vi "ConfigureRF.vi"(8 "error in (no error)":errorcluster, 11 "reference in":refnum<class "niMmWave_Reciever.lvclass">) -> (0 "error out":errorcluster, 3 "reference out":refnum<class "niMmWave_Reciever.lvclass">)   [LabVIEW 2019, in "niMmWave_Reciever.lvclass"]
doc: "Configures RF setting at specified port:\n<b>Frequency</b> - operating frequency (RF/IF)\n<b>Gain</b> - Signal gain"
uses:
  niMmWave_Reciever.lvclass
  C:/Barkhausen mmWave radar/Development/modules/mmw_instrument/src_LabVIEW/Host/SubVIs/mmWave instrument_class/mmWave instrument.lvclass
  Low-level/TypeDefs/Front End Configuration.ctl
  Low-level/TypeDefs/Channel Configuration.ctl
  <instrlib>/niMmWave/ni3620/Config/v1/Host/Public/Typedefs/mmWave Port.ctl
  mmWave instrument_class/mmWave instrument.lvclass
  mmWave HW Control/mmWave HW Control.lvlib
  <instrlib>/niMmWave/ni3620/Config/v1/Host/niMmWave Config v1 Host.lvlib
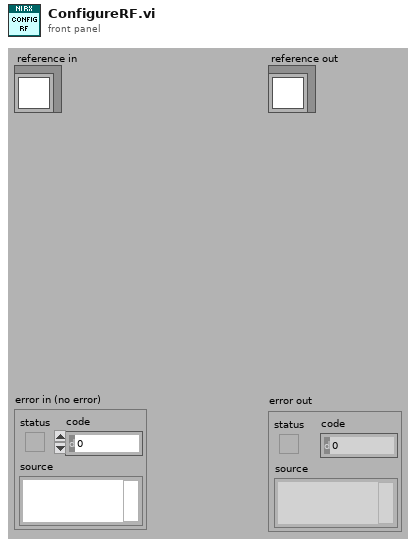
[diagram p1: front panel]
types:
  T1 = typedef "niMmWave Config v1 Host.lvlib/mmWave Port.ctl" = string
  T2 = typedef "Front End Configuration.ctl" = cluster{"port select":enum16{"IF Port", "Loopback", "Sync Port"}, "Rx hardware configuration":T3, "Tx hardware configuration":T3}
  T3 = typedef "Channel Configuration.ctl" = cluster{"gain (dB)":dbl, "frequency (Hz)":dbl, "mmWave adapter":string, "adapter active port":T1}
  T4 = typedef "niMmWave_Reciever.lvclass/ObjectAttributesRef.ctl" = refnum<data-value>
  T5 = typedef "mmWave instrument.lvclass/ObjectAttributes.ctl" = cluster{"mode":T6, "instr state":T7, "Max Fs":dbl, "Equalization coeff":cdb[], "LO sync en":bool, "Trig sync en":bool, "LO sources":T8, "LO Export":T9, "Fc.range":cluster{"min":dbl, "max":dbl}, "Sync mode":T10, "equalization en":bool, "sequence":string[]}
  T6 = typedef "mmWave instrument.lvclass/Instrument mode.ctl" = enum16{"RF", "IF", "BB"}
  T7 = typedef "mmWave instrument.lvclass/Instrument state.ctl" = enum16{"Off", "Initialization", "Configuration", "Running", "Calibration"}
  T8 = typedef "mmWave HW Control.lvlib/LO sources.ctl" = cluster{"RX/LO1 src":string, "TX/LO1 src":string, "LO2 src":string}
  T9 = typedef "mmWave HW Control.lvlib/LO export.ctl" = cluster{"TX LO1 export":bool, "TX LO1 export level":dbl, "RX LO1 export":bool, "RX LO1 export level":dbl, "LO2 export":bool, "LO2 export level":dbl}
  T10 = typedef "mmWave instrument.lvclass/Sync mode.ctl" = enum16{"Slave", "Master"}
  T11 = typedef "niMmWave_Reciever.lvclass/ObjectAttributes.ctl" = cluster{"session":T12[], "HW.RX devices":T26, "RF config":T27, "RX trigger options":T28, "RX samples":i32, "RX Fs":dbl}
  T12 = typedef "Session.ctl" = cluster{"3620 session":refnum<queue>, "tx baseband session":T13, "rx baseband session":T21, "tx gain (dB)":dbl, "rx gain (dB)":dbl, "hardware configuration":T22, "gain ranging":T24[], "pxi trigger bus information":T25}
  T13 = typedef "Tx Baseband Session.ctl" = cluster{"3610 session":T14, "7902 reference":T20}
  T14 = typedef "ni3610_and_ni3630_Driver_Lib.lvlib/Main Settings.ctl" = cluster{"VISA resource name":refnum<visa-resource-name>, "Address Space":T15, "window_offset":u32, "register_addresses":T16, "required_MM_fpga_version":cluster{"signature":u32, "hardware":u32, "current revision":u32, "oldest revision":u32}, "CPLD Oldest Compat Version ":cluster{"hardware":u32, "CPLD firmware":u32}, "MM_FPGA_image_location":string, "is_init":bool, "card_type":T17, "DacLmkConfigFileName":string, "AdcLmkConfigFileName":string, "AdcConfigFileName":string, "DacConfigFileName_RevA":string, "DacConfigFileName_RevB":string, "Mulde hardware revision":u8, "bypass DAC PLL\n":bool, "IQ Card Revision":T18, "board capability":T19}
  T15 = typedef "VISA Register Access Address Space.ctl" = u16
  T16 = typedef "ni3610_and_ni3630_Driver_Lib.lvlib/Register Adresses.ctl" = cluster{"MM based Registers":cluster{"Revision":u32, "OldestCompatRev":u32, "signature":u32, "scratch":u32, "LedControl":u32, "BoardHwRev":u32, "BoardControl":u32, "ThermalStatus":u32, "BasebandStatus":u32, "BasebandControl":u32, "BasebandAuxSetup":u32, "BasebandAuxStatus":u32, "LmkSyncOutSetup":u32, " AdcSyncOutSetup":u32, " InjSyncOutSetup":u32, " PxiTrig0OutSetup":u32, " PxiTrig1OutSetup":u32, " PxiTrig2OutSetup":u32, " PxiTrig3OutSetup":u32, " PxiTrig4OutSetup":u32, " PxiTrig5OutSetup":u32, " PxiTrig6OutSetup":u32, " PxiTrig7OutSetup":u32}, "CPLD based Registers":cluster{"SlaveSignature":u32, "SlaveRevision":u32, "SlaveOldestCompatRev":u32, "SlaveScratch":u32, "SlaveSetup":u32, "SlaveStatus":u32, "IDacReg_offset":u32, "LMKRegGrp0_offset":u32, "QDacReg_offset":u32, "BrdTempSensorVal":u32, "TempSensorPowerDown":u32, "GPIOReg_offset":u32, "IAdcReg_offset":u32, "QAdcReg_offset":u32, "LMKRegGrp1_offset":u32, "QadcTempSensorVal":u32, "IadcTempSensorVal":u32, "RevisionReg":u32, "VcxoReg":u32, "CpldStatusReg":u32, "PowerReg":u32, "VBiasEnReg":u32, "ExtRefOeReg":u32, "QdacCtrlReg":u32, "QdacStatusReg":u32, "IdacCtrlReg":u32, "IdacStatusReg":u32, "QdacJtagIn":u32, "QdacJtagOut":u32, "IdacJtagIn":u32, "IdacJtagOut":u32, "IqDcSetupReg":u32, "QadcStatusReg":u32, "IadcStatusReg":u32, "BrdSetupReg":u32, "IqDcRevisionReg":u32, "PllStatusReg":u32, "EndpointScratchReg":u32, "AdcSyncCfgReg":u32, "IqCardOpampReg":u32}, "CPLD Register Offset":u32, "MM  Register Offset":u32, " PxiTrig0OutSetup":u32}
  T17 = typedef "ni3610_and_ni3630_Driver_Lib.lvlib/Base Card Type.ctl" = enum16{"unspecified", "ADC", "DAC"}
  T18 = typedef "ni3610_and_ni3630_Driver_Lib.lvlib/IQ Card Revision.ctl" = enum16{"RevA", "RevB", "RevC", "RevD"}
  T19 = typedef "ni3610_and_ni3630_Driver_Lib.lvlib/Board Capability.ctl" = cluster{"baseband sync":enum16{"no baseband sync", "baseband sync"}}
  T20 = typedef "Blank FPGA Reference.ctl" = refnum<k20>
  T21 = typedef "Rx Baseband Session.ctl" = cluster{"3630 session":T14, "7902 reference":T20}
  T22 = typedef "Hardware Configuration.ctl" = cluster{"direction":T23, "baseband only":bool}
  T23 = typedef "Direction.ctl" = enum16{"Transceiver", "Receiver", "Transmitter"}
  T24 = typedef "Gain Ranging.ctl" = cluster{"gain ranging active scope":string, "gain ranging stream session":refnum<k20>}
  T25 = typedef "PXI Trigger Bus Info.ctl" = cluster{"chassis resource name":refnum<visa-resource-name>, "7902R (TX)":i16, "3610 (TX)":i16, "3620 (IF)":i16, "3630 (RX)":i16, "7902R (RX)":i16}
  T26 = typedef "mmWave HW Control.lvlib/HW RX resources cluster.ctl" = cluster{"HW.IF":tag, "HW.ADC":refnum<visa-resource-name>, "HW.RX FPGA":tag}
  T27 = typedef "mmWave HW Control.lvlib/HW RX RF config cluster.ctl" = cluster{"Gain":dbl, "Frequency":dbl, "mmWave adapter":string}
  T28 = typedef "TX trigger config.ctl" = cluster{"delay":dbl, "trig source":T29, "PXI src":i32, "export":T30, "PXI dest":i32}
  T29 = typedef "FPGA Utility.lvlib/FPGA driver trigger source.ctl" = enum16{"Use Tclk", "PXI_Trig", "Aurora RX trig"}
  T30 = typedef "FPGA Utility.lvlib/FPGA driver trigger destination.ctl" = enum16{"None", "Source trig", "Synced trig", "Delayed sync"}
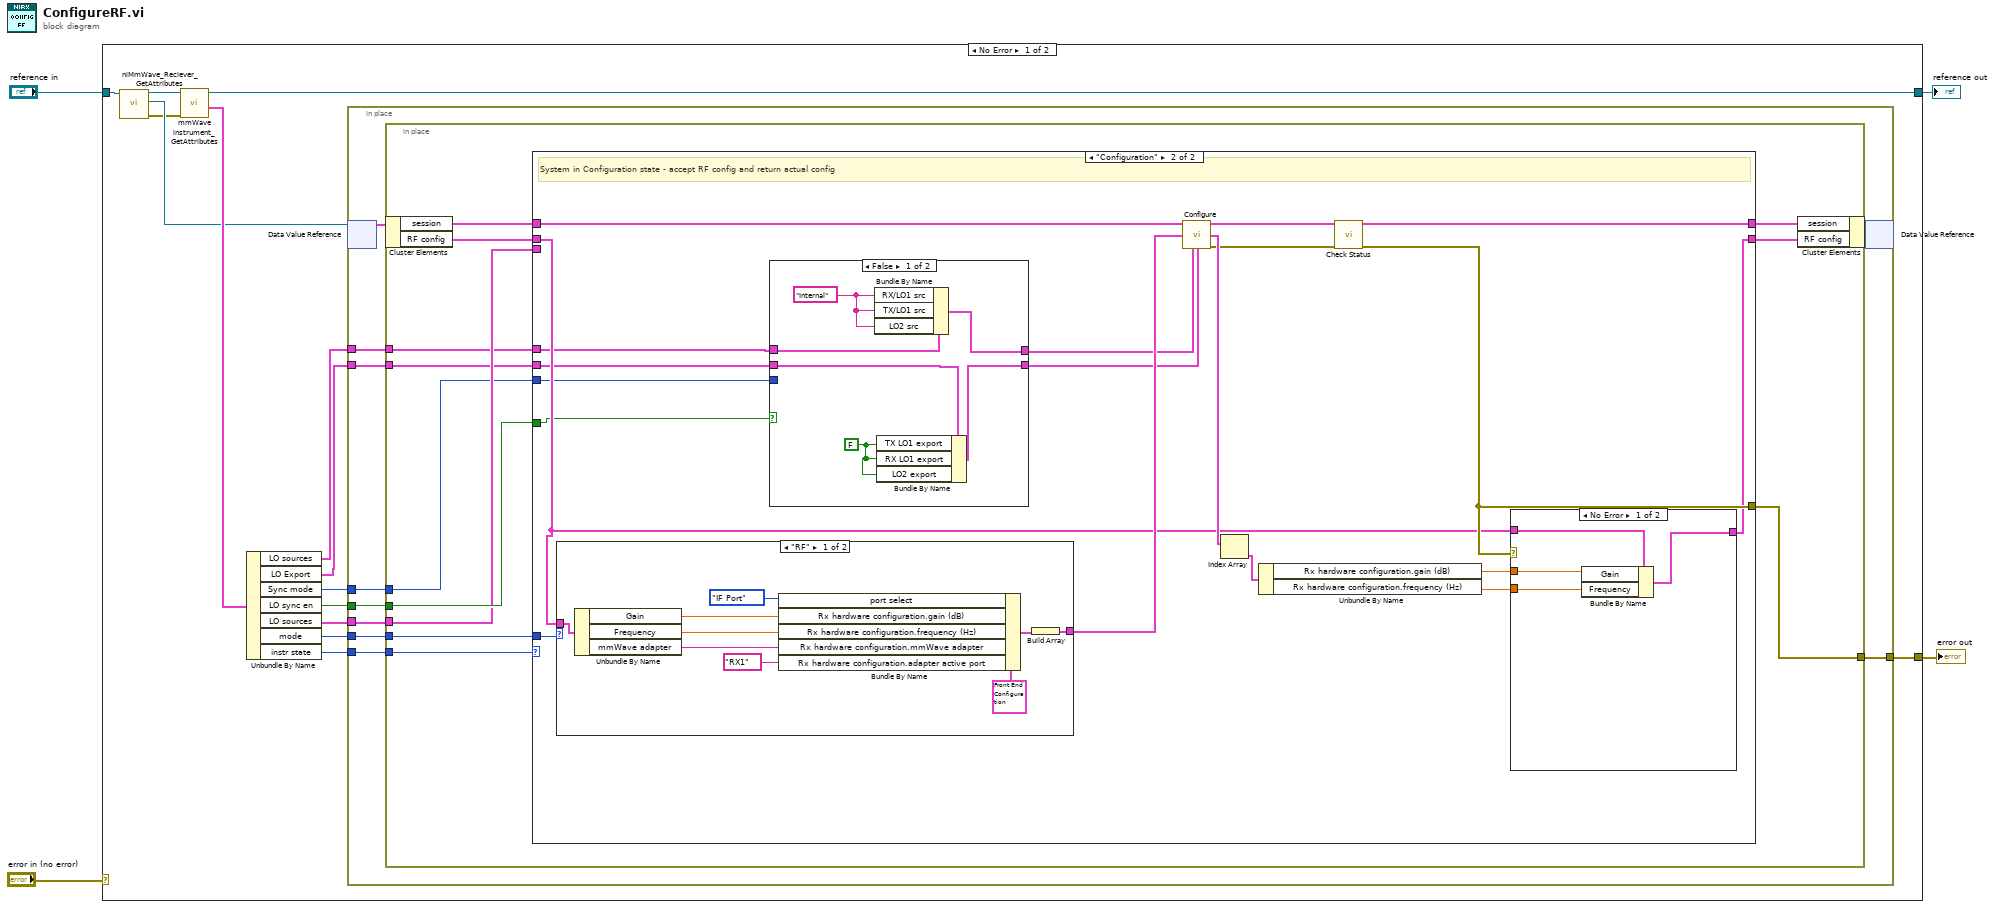
[diagram p0: block diagram]
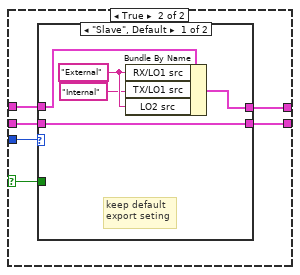
[diagram p3: hidden frame]
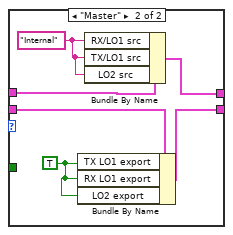
[diagram p4: hidden frame]
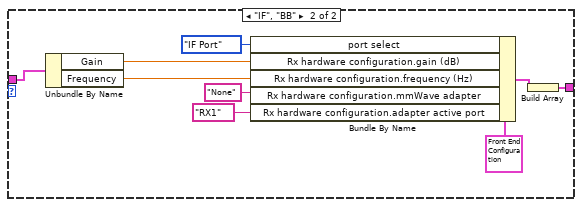
[diagram p6: hidden frame]
diagram:
  n1 = case shown="No Error" "error in (no error)" {
    selector: "error in (no error)" -> [_ w109]
    tunnel: [w12 w109] -> w3
    tunnel: [w16 w108] -> w1
    tunnel: "reference in" -> [w17 w108]
    frame No Error {
      n2 = call "niMmWave_Reciever_GetAttributes.vi"("reference in"=w17) -> ("error out"=w13:errorcluster, "attributes ref"=w14:T4, "reference out"=w18:refnum<class "niMmWave_Reciever.lvclass">)  [unwired: 7 in, 1 out]
      n3 = call "mmWave instrument_GetAttributes.vi"("error in (no error)"=w13, "reference in"=w18) -> ("attributes"=w15:T5, "reference out"=w16:refnum<class "niMmWave_Reciever.lvclass">)  [unwired: 6 in, 2 out]
      n4 = Unbundle By Name(w15) -> ("LO sources"=w7:T8, "LO Export"=w6:T9, "Sync mode"=w5:T10, "LO sync en"=w9:bool, "LO sources"=w8:T8, "mode"=w11:T6, "instr state"=w10:T7)
      n5 = in-place {
        in-place-border: [w27] -> w12
        in-place-border: w11 -> [w26]
        in-place-border: w10 -> [w25]
        in-place-border: w9 -> [w23]
        in-place-border: w8 -> [w22]
        in-place-border: w7 -> [w21]
        in-place-border: w6 -> [w20]
        in-place-border: w5 -> [w19]
        n6 = in-place-dvr #1(w14) -> (w24:T11)  [unwired: 1 out]
        n7 = in-place {
          in-place-border: [w37] -> w27
          in-place-border: w26 -> [w38]
          in-place-border: w25 -> [w35]
          in-place-border: w23 -> [w33]
          in-place-border: w22 -> [w32]
          in-place-border: w21 -> [w31]
          in-place-border: w20 -> [w30]
          in-place-border: w19 -> [w29]
          n8 = in-place-cluster #2(w24) -> ("session"=w40:T12[], "RF config"=w34:T27)
          n9 = case shown="\"Configuration\"" w35 {
            tunnel: w40 -> [w42 w60]
            tunnel: [w42 w59] -> w39
            tunnel: w38 -> [_ w58]
            tunnel: [_ w55] -> w37
            tunnel: [w41 w52] -> w36
            tunnel: w34 -> [w41 w51]
            tunnel: w33 -> [_ w46]
            tunnel: w32 -> [_ _]
            tunnel: w31 -> [_ w47]
            tunnel: w30 -> [_ w45]
            tunnel: w29 -> [_ w43]
            frame "Off", Default {
            }
            frame "Configuration" {
              # "System in Configuration state - accept RF config and return actual config"
              n10 = case shown="\"RF\"" w58 {
                tunnel: [w98 w107] -> w61
                tunnel: w51 -> [w93 w102]
                frame "RF" {
                  n11 = Unbundle By Name(w93) -> ("Gain"=w92:dbl, "Frequency"=w91:dbl, "mmWave adapter"=w90:string)
                  n12 = Bundle By Name(cluster=T2 {"port select"=enum."Loopback", "Rx hardware configuration"={"gain (dB)"=15.0, "frequency (Hz)"=12000000000.0, "mmWave adapter"="None", "adapter active port"=""}, "Tx hardware configuration"={"gain (dB)"=-15.0, "frequency (Hz)"=12000000000.0, "mmWave adapter"="None", "adapter active port"=""}} ("device configuration [channel]"), "port select"=enum16{"IF Port", "Loopback", "Sync Port"}."IF Port", "Rx hardware configuration.gain (dB)"=w92, "Rx hardware configuration.frequency (Hz)"=w91, "Rx hardware configuration.mmWave adapter"=w90, "Rx hardware configuration.adapter active port"=T1 "RX1") -> (w97:T2)
                  n13 = Build Array(w97) -> (w98:T2[])
                }
                frame "IF", "BB" {
                  n14 = Unbundle By Name(w102) -> ("Gain"=w101:dbl, "Frequency"=w100:dbl)
                  n15 = Bundle By Name(cluster=T2 {"port select"=enum."Loopback", "Rx hardware configuration"={"gain (dB)"=15.0, "frequency (Hz)"=12000000000.0, "mmWave adapter"="None", "adapter active port"=""}, "Tx hardware configuration"={"gain (dB)"=-15.0, "frequency (Hz)"=12000000000.0, "mmWave adapter"="None", "adapter active port"=""}} ("device configuration [channel]"), "port select"=enum16{"IF Port", "Loopback", "Sync Port"}."IF Port", "Rx hardware configuration.gain (dB)"=w101, "Rx hardware configuration.frequency (Hz)"=w100, "Rx hardware configuration.mmWave adapter"="None", "Rx hardware configuration.adapter active port"=T1 "RX1") -> (w106:T2)
                  n16 = Build Array(w106) -> (w107:T2[])
                }
              }
              n17 = case shown="False" w46 {
                selector: w46 -> [_ w68]
                tunnel: w47 -> [w67 w69]
                tunnel: w45 -> [w63 w73]
                tunnel: [w66 w70] -> w48
                tunnel: [w62 w72] -> w44
                tunnel: w43 -> [_ w71]
                frame False {
                  w64 = FALSE
                  w65 = "Internal" ("RX/LO1 src")
                  n18 = Bundle By Name(cluster=w67, "RX/LO1 src"=w65, "TX/LO1 src"=w65, "LO2 src"=w65) -> (w66:T8)
                  n19 = Bundle By Name(cluster=w63, "TX LO1 export"=w64, "RX LO1 export"=w64, "LO2 export"=w64) -> (w62:T9)
                }
                frame True {
                  n20 = case shown="\"Slave\", Default" w71 {
                    tunnel: w73 -> [w75 w84]
                    tunnel: [w75 w83] -> w72
                    tunnel: [w77 w80] -> w70
                    tunnel: w69 -> [w78 w81]
                    tunnel: w68 -> [_ _]
                    frame "Slave", Default {
                      w76 = "External" ("RX/LO1 src")
                      # "keep default\nexport seting"
                      n21 = Bundle By Name(cluster=w78, "RX/LO1 src"=w76, "TX/LO1 src"="Internal" ("RX/LO1 src"), "LO2 src"=w76) -> (w77:T8)
                    }
                    frame "Master" {
                      w79 = "Internal" ("RX/LO1 src")
                      w82 = TRUE
                      n22 = Bundle By Name(cluster=w84, "TX LO1 export"=w82, "RX LO1 export"=w82, "LO2 export"=w82) -> (w83:T9)
                      n23 = Bundle By Name(cluster=w81, "RX/LO1 src"=w79, "TX/LO1 src"=w79, "LO2 src"=w79) -> (w80:T8)
                    }
                  }
                }
              }
              n24 = call "Configure.vi"("session in"=w60, "device configuration [channel]"=w61, "LO sources"=w48, "LO Export"=w44) -> ("session out"=w50:T12[], "coerced device configuration [channel]"=w57:T2[], "error out"=w49:errorcluster)  [unwired: 9 in]
              n25 = Index Array(array=w57) -> (element=w56:T2)  [unwired: 1 in]
              n26 = Unbundle By Name(w56) -> ("Rx hardware configuration.gain (dB)"=w54:dbl, "Rx hardware configuration.frequency (Hz)"=w53:dbl)
              n27 = call "Check Status.vi"("session in"=w50, "error in"=w49) -> ("session out"=w59:T12[], "error out"=w55:errorcluster)  [unwired: 9 in, 3 out]
              n28 = case shown="No Error" w55 {
                tunnel: w51 -> [w88 w89]
                tunnel: w54 -> [w86 _]
                tunnel: w53 -> [w85 _]
                tunnel: [w87 w89] -> w52
                frame No Error {
                  n29 = Bundle By Name(cluster=w88, "Gain"=w86, "Frequency"=w85) -> (w87:T27)
                }
                frame Error {
                }
              }
            }
          }
          n30 = in-place-cluster #2("session"=w39, "RF config"=w36) -> (w28:T11)
        }
        n31 = in-place-dvr #1(w28) -> ()  [unwired: 2 out]
      }
    }
    frame Error {
    }
  }
  "error out" <- w3
  "reference out" <- w1
